vi "OxITC503 _Utility_ Talk.vi"(0 "VISA session":refnum<visa-resource-name>, 2 "Command":string, 3 "error in (no error)":errorcluster, 4 "timeout (5000)":u32=5000) -> (5 "VISA session":refnum<visa-resource-name>, 6 "read buffer":string, 7 "error out (no error)":errorcluster)   [LabVIEW 2014]
doc: "This VI allows an application to communicate with an Oxford Instruments ITC 503 using LabVIEW's VISA API.\n\nSends a command to the ITC503. If the device sends a return message it is stored in the \"read buffer\" output. Otherwise the buffer is returned empty."
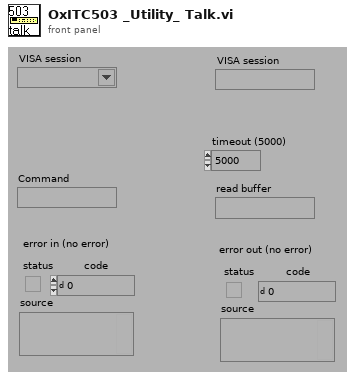
[diagram p1: front panel]
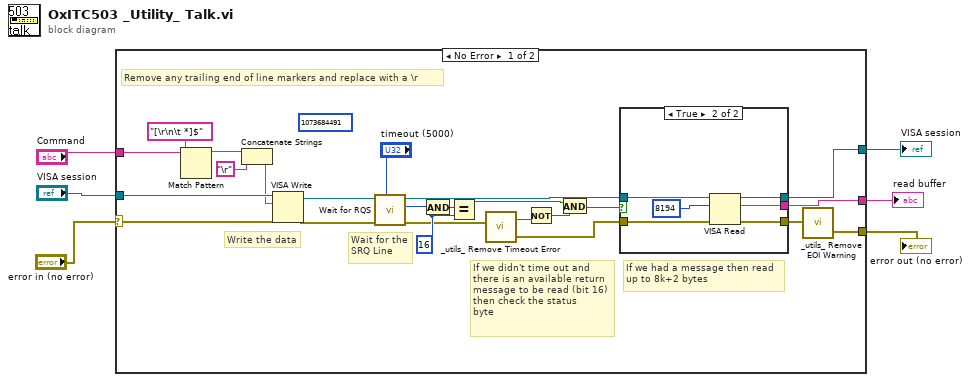
[diagram p0: block diagram]
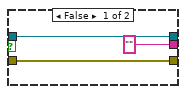
[diagram p2: hidden frame]
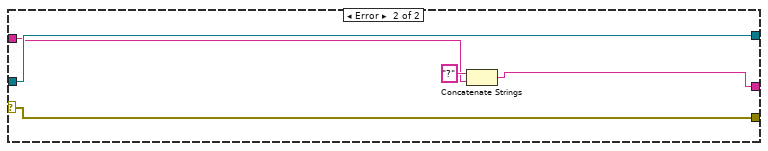
[diagram p3: hidden frame]
diagram:
  n1 = case shown="No Error" "error in (no error)" {
    selector: "error in (no error)" -> [w7 w44]
    tunnel: [w30 w40] -> w6
    tunnel: "Command" -> [w29 w41]
    tunnel: "VISA session" -> [w28 w43]
    tunnel: [w27 w44] -> w3
    tunnel: [w26 w43] -> w2
    frame No Error {
      w15 = u16 16 ("y")
      (unwired) u32 1073684491 ("event type")
      # "If we had a message then read\nup to 8k+2 bytes"
      # "If we didn't time out and\nthere is an available return\nmessage to be read (bit 16)\nthen check the status\nbyte"
      # "Wait for the\nSRQ Line"
      # "Write the data"
      # "Remove any trailing end of line markers and replace with a \\r"
      n2 = Match Pattern(string=w29, regular expression="[\r\n\t *]$") -> (before substring=w23:string)  [unwired: 1 in, 3 out]
      n3 = Concatenate Strings(w23, "\r") -> (w25:string)
      n4 = VISA Write(VISA resource name=w28, write buffer=w25, error in (no error)=w7) -> (VISA resource name out=w19:refnum<visa-resource-name>, error out=w20:errorcluster)  [unwired: 1 out]
      n5 = call <vilib>:"Wait for RQS.VI"("timeout (25000 ms)"="timeout (5000)", "error in (no error)"=w20, "VISA resource name"=w19) -> ("error out"=w13:errorcluster, "status byte"=w17:u16, "VISA resource name out"=w14:refnum<visa-resource-name>)  [unwired: 6 in]
      n6 = And(x=w17, y=w15) -> (x .and. y?=w16:u16)
      n7 = Equal?(x=w16, y=w15) -> (x = y?=w11:bool)
      n8 = call "_utils_ Remove Timeout Error.vi"("error in"=w13) -> ("Operation timed out?"=w10:bool, "error out"=w12:errorcluster)
      n9 = Not(x=w10) -> (.not. x?=w9:bool)
      n10 = And(x=w11, y=w9) -> (x .and. y?=w8:bool)
      n11 = case shown="True" w8 {
        tunnel: w14 -> [w32 w39]
        tunnel: w12 -> [w33 w38]
        tunnel: [w33 w36] -> w21
        tunnel: [w32 w37] -> w26
        tunnel: ["" ("read buffer") w35] -> w30
        frame False {
        }
        frame True {
          n12 = VISA Read(VISA resource name=w39, byte count=u32 8194 ("byte count (0)"), error in (no error)=w38) -> (VISA resource name out=w37:refnum<visa-resource-name>, read buffer=w35:string, error out=w36:errorcluster)  [unwired: 1 out]
        }
      }
      n13 = call "_utils_ Remove EOI Warning.vi"("error in"=w21) -> ("error out"=w27:errorcluster)  [unwired: 1 out]
    }
    frame Error {
      n14 = Concatenate Strings("?" ("string"), w41) -> (w40:string)
    }
  }
  "read buffer" <- w6
  "error out (no error)" <- w3
  "VISA session" <- w2
